vi "CH_LM App FGV DAQStatus.vi"(7 "Function":T2=enum."get", 8 "error in (no error)":errorcluster, 9 "DAQ Status":T1={"Command"="", "Collection Mode"=enum."Streaming", "T / ms"=1, "Sample Collection"=enum."Continuous", "Sample Size"=100, "Pause"=FALSE} {"Sample Size" min=1}, 11 "VI Ref":refnum<vi>) -> (0 "error out":errorcluster, 1 "DAQ Status":T1={"Command"="", "Collection Mode"=enum."Streaming", "T / ms"=1, "Sample Collection"=enum."Continuous", "Sample Size"=100, "Pause"=FALSE} {"Sample Size" min=1}, 3 "VI Ref":refnum<vi>, 4 "DAQ Status Array":T1[](array[typedef]) {"Sample Size" min=1}, 6 "empty":bool)   [LabVIEW 2012, in "CH_LM App.lvlib"]
doc: "This functional global variable maintains the Status of all LabMax DAQ threads."
uses:
  CH_LM App.lvlib
  CH_LM.lvlib
  CH_LM App DAQ Status.ctl
  _CH_LM/CH_LM FGV Functions.ctl
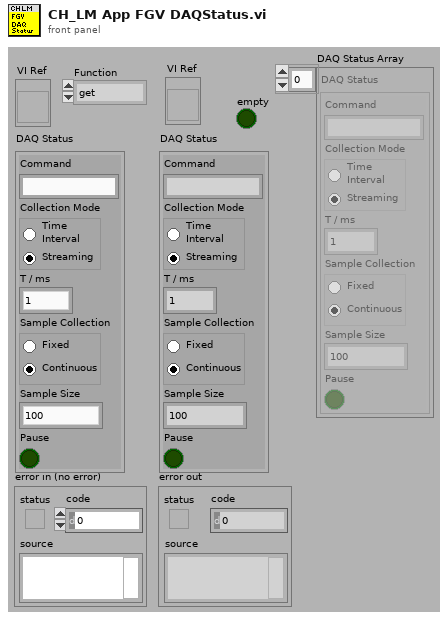
[diagram p1: front panel]
types:
  T1 = typedef "CH_LM App.lvlib/CH_LM App DAQ Status.ctl" = cluster{"Command":string, "Collection Mode":enum32{"Time\nInterval", "Streaming"}, "T / ms":i32, "Sample Collection":enum32{"Fixed", "Continuous"}, "Sample Size":i32, "Pause":bool}
  T2 = typedef "CH_LM.lvlib/CH_LM FGV Functions.ctl" = enum16{"create", "get", "set", "remove", "clear", "getBySerial"}
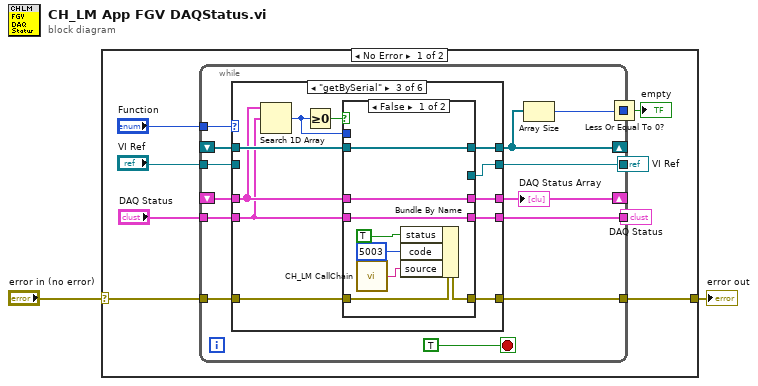
[diagram p0: block diagram]
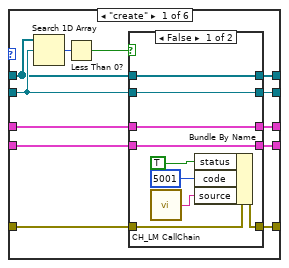
[diagram p2: hidden frame]
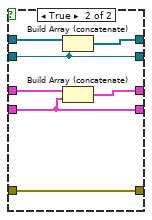
[diagram p3: hidden frame]
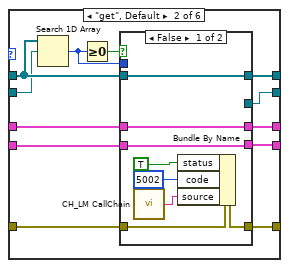
[diagram p4: hidden frame]
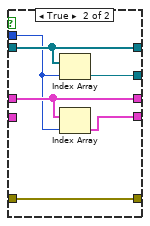
[diagram p5: hidden frame]
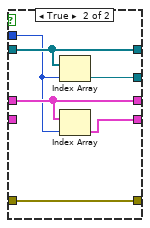
[diagram p6: hidden frame]
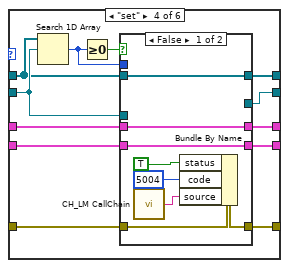
[diagram p7: hidden frame]
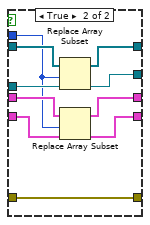
[diagram p8: hidden frame]
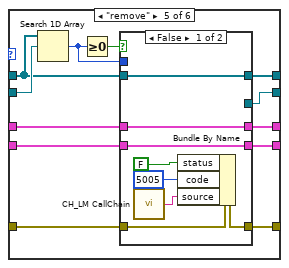
[diagram p9: hidden frame]
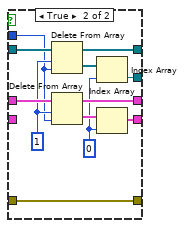
[diagram p10: hidden frame]
diagram:
  n1 = case shown="No Error" "error in (no error)" {
    selector: "error in (no error)" -> [w10 w167]
    tunnel: [w9 w167] -> w1
    frame No Error {
      n2 = while {
        tunnel: "Function" -> [w23]
        shift-right: [w12] -> _
        shift-left: _ -> [w21]
        tunnel: "VI Ref" -> [w22]
        tunnel: [w20] -> w5
        tunnel: w10 -> [w19]
        tunnel: [w18] -> w9
        shift-right: [w16] -> _
        shift-left: _ -> [w15]
        tunnel: "DAQ Status" -> [w17]
        tunnel: [w14] -> w7
        tunnel: [w13] -> w4
        stop <- TRUE stop-if-true
        n3 = case shown="\"getBySerial\"" w23 {
          tunnel: w22 -> [w27 w54 _ w105 w134 _]
          tunnel: w21 -> [w26 w55 w89 w104 w133 w165]
          tunnel: [w36 w60 w84 w110 w138 w165] -> w12
          tunnel: [w34 w59 w83 w115 w143 _] -> w20
          tunnel: w19 -> [w33 w62 w86 w112 w140 w166]
          tunnel: [w32 w61 w85 w111 w139 w166] -> w18
          tunnel: w17 -> [w31 w53 w79 w107 w132 w164]
          tunnel: [w30 w57 w82 w108 w136 _] -> w16
          tunnel: w15 -> [w29 w58 w80 w109 w137 _]
          tunnel: [w28 w56 w81 w106 w135 w164] -> w14
          frame "create" {
            n4 = Search 1D Array(1D array=w26, element=w27) -> (index of element=w35:i32)  [unwired: 1 out]
            n5 = Less Than 0?(x=w35) -> (x < 0?=w25:bool)
            n6 = case shown="False" w25 {
              tunnel: w27 -> [w44 w50]
              tunnel: w26 -> [w45 w52]
              tunnel: [w45 w51] -> w36
              tunnel: [w44 w50] -> w34
              tunnel: w33 -> [w43 w49]
              tunnel: [w42 w49] -> w32
              tunnel: w31 -> [w37 w46]
              tunnel: [w38 w48] -> w30
              tunnel: w29 -> [w38 w47]
              tunnel: [w37 w46] -> w28
              frame False {
                n7 = call "CH_LM CallChain.vi"() -> ("ChallChain"=w39:string)
                n8 = Bundle By Name(cluster=w43, "status"=TRUE, "code"=5001, "source"=w39) -> (w42:errorcluster)
              }
              frame True {
                n9 = Build Array (concatenate)(w52, w50) -> (w51:refnum<vi>[])
                n10 = Build Array (concatenate)(w47, w46) -> (w48:T1[])
              }
            }
          }
          frame "get", Default {
            n11 = Search 1D Array(1D array=w55, element=w54) -> (index of element=w64:i32)  [unwired: 1 out]
            n12 = Greater Or Equal To 0?(x=w64) -> (x >= 0?=w63:bool)
            n13 = case shown="False" w63 {
              tunnel: w55 -> [w67 w76]
              tunnel: [_ w78] -> w59
              tunnel: w64 -> [_ w73]
              tunnel: w62 -> [w69 w77]
              tunnel: [w68 w77] -> w61
              tunnel: [w67 w76] -> w60
              tunnel: w58 -> [w66 w75]
              tunnel: [w66 w75] -> w57
              tunnel: [w65 w74] -> w56
              tunnel: w53 -> [w65 _]
              frame False {
                n14 = call "CH_LM CallChain.vi"() -> ("ChallChain"=w70:string)
                n15 = Bundle By Name(cluster=w69, "status"=TRUE, "code"=5002, "source"=w70) -> (w68:errorcluster)
              }
              frame True {
                n16 = Index Array(array=w76, index=w73) -> (element=w78:refnum<vi>)
                n17 = Index Array(array=w75, index=w73) -> (element=w74:T1)
              }
            }
          }
          frame "getBySerial" {
            n18 = Search 1D Array(1D array=w80, element=w79) -> (index of element=w88:i32)  [unwired: 1 out]
            n19 = Greater Or Equal To 0?(x=w88) -> (x >= 0?=w87:bool)
            n20 = case shown="False" w87 {
              tunnel: w89 -> [w92 w101]
              tunnel: [_ w103] -> w83
              tunnel: w88 -> [_ w98]
              tunnel: w86 -> [w94 w102]
              tunnel: [w93 w102] -> w85
              tunnel: [w92 w101] -> w84
              tunnel: w80 -> [w91 w100]
              tunnel: [w91 w100] -> w82
              tunnel: [w90 w99] -> w81
              tunnel: w79 -> [w90 _]
              frame False {
                n21 = call "CH_LM CallChain.vi"() -> ("ChallChain"=w95:string)
                n22 = Bundle By Name(cluster=w94, "status"=TRUE, "code"=5003, "source"=w95) -> (w93:errorcluster)
              }
              frame True {
                n23 = Index Array(array=w101, index=w98) -> (element=w103:refnum<vi>)
                n24 = Index Array(array=w100, index=w98) -> (element=w99:T1)
              }
            }
          }
          frame "set" {
            n25 = Search 1D Array(1D array=w104, element=w105) -> (index of element=w114:i32)  [unwired: 1 out]
            n26 = Greater Or Equal To 0?(x=w114) -> (x >= 0?=w113:bool)
            n27 = case shown="False" w113 {
              tunnel: w104 -> [w118 w129]
              tunnel: [_ w130] -> w115
              tunnel: w114 -> [_ w124]
              tunnel: w112 -> [w120 w131]
              tunnel: [w119 w131] -> w111
              tunnel: [w118 w128] -> w110
              tunnel: w105 -> [_ w130]
              tunnel: w109 -> [w117 w127]
              tunnel: [w117 w126] -> w108
              tunnel: w107 -> [w116 w125]
              tunnel: [w116 w125] -> w106
              frame False {
                n28 = call "CH_LM CallChain.vi"() -> ("ChallChain"=w121:string)
                n29 = Bundle By Name(cluster=w120, "status"=TRUE, "code"=5004, "source"=w121) -> (w119:errorcluster)
              }
              frame True {
                n30 = Replace Array Subset(array=w129, new element=w130, index=w124) -> (w128:refnum<vi>[])
                n31 = Replace Array Subset(array=w127, new element=w125, index=w124) -> (w126:T1[])
              }
            }
          }
          frame "remove" {
            n32 = Search 1D Array(1D array=w133, element=w134) -> (index of element=w142:i32)  [unwired: 1 out]
            n33 = Greater Or Equal To 0?(x=w142) -> (x >= 0?=w141:bool)
            n34 = case shown="False" w141 {
              tunnel: w133 -> [w146 w162]
              tunnel: [_ w160] -> w143
              tunnel: w142 -> [_ w153]
              tunnel: w140 -> [w148 w163]
              tunnel: [w147 w163] -> w139
              tunnel: [w146 w161] -> w138
              tunnel: w137 -> [w145 w157]
              tunnel: [w145 w156] -> w136
              tunnel: [w144 w155] -> w135
              tunnel: w132 -> [w144 _]
              frame False {
                n35 = call "CH_LM CallChain.vi"() -> ("ChallChain"=w149:string)
                n36 = Bundle By Name(cluster=w148, "status"=FALSE, "code"=5005, "source"=w149) -> (w147:errorcluster)
              }
              frame True {
                w152 = 0 ("index")
                w154 = 1 ("length")
                n37 = Delete From Array(array=w162, length=w154, index=w153) -> (deleted portion=w159:refnum<vi>[], array with subset deleted=w161:refnum<vi>[])
                n38 = Delete From Array(array=w157, length=w154, index=w153) -> (deleted portion=w158:T1[], array with subset deleted=w156:T1[])
                n39 = Index Array(array=w159, index=w152) -> (element=w160:refnum<vi>)
                n40 = Index Array(array=w158, index=w152) -> (element=w155:T1)
              }
            }
          }
          frame "clear" {
          }
        }
        "DAQ Status Array" <- w16
        n41 = Array Size(array=w12) -> (size(s)=w13:i32)
      }
      "DAQ Status" <- w7
      "VI Ref" <- w5
      n42 = Less Or Equal To 0?(x=w4) -> (x <= 0?=→"empty":bool)
    }
    frame Error {
    }
  }
  "error out" <- w1
